vi "isHomeCheckFGV.vi"(10 "isHomeCheck?":bool=TRUE, 11 "state":enum16{"get", "set"}(ring)) -> (3 "HomeisCheck":bool)   [LabVIEW 2020]
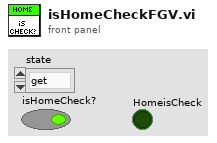
[diagram p1: front panel]
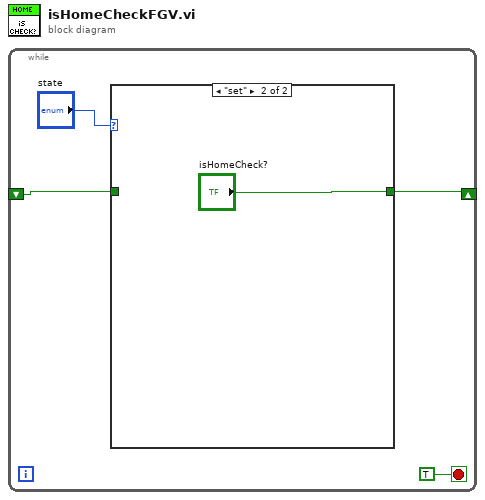
[diagram p0: block diagram]
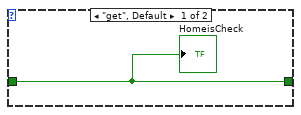
[diagram p2: hidden frame]
diagram:
  n1 = while {
    shift-right: [w3] -> _
    shift-left: _ -> [w2]
    stop <- TRUE stop-if-true
    n2 = case shown="\"set\"" "state" {
      tunnel: [w5 "isHomeCheck?"] -> w3
      tunnel: w2 -> [w5 _]
      frame "get", Default {
        "HomeisCheck" <- w5
      }
      frame "set" {
      }
    }
  }
